vi "ECSv1_12.vi"() -> ()   [LabVIEW 2018]
uses:
  <vilib>/sound2/lvsound2.llb/Sampling Mode.ctl
  <vilib>/sound2/lvsound2.llb/Sound Data Format.ctl
  <vilib>/DAQmx/write.llb/DAQmx Write (Analog 1D DBL 1Chan NSamp).vi
  <vilib>/DAQmx/write.llb/DAQmx Write (Analog Wfm 1Chan NSamp).vi
  <vilib>/DAQmx/write.llb/DAQmx Write (Digital Bool 1Line 1Point).vi
  <vilib>/DAQmx/read.llb/DAQmx Read (Analog 1D Wfm NChan NSamp).vi
  <vilib>/DAQmx/create/channels.llb/DAQmx Create Channel (AI-Voltage-Basic).vi
  <vilib>/DAQmx/configure/timing.llb/DAQmx Timing (Sample Clock).vi
  <vilib>/sound2/lvsound2.llb/Sound File Write Open.vi
  <vilib>/sound2/lvsound2.llb/Sound Input Read (DBL).vi
  <vilib>/measure/maspectr.llb/FFT Power Spectral Density for N Chan.vi
  <vilib>/sound2/lvsound2.llb/Sound File Write (DBL).vi
  <vilib>/DAQmx/create/channels.llb/DAQmx Create Channel (DO-Digital Output).vi
  <vilib>/DAQmx/miscellaneous.llb/DAQmx Fill In Error Info.vi
  <vilib>/DAQmx/create/channels.llb/DAQmx Create Channel (CO-Pulse Generation-Time).vi
  <vilib>/DAQmx/configure/timing.llb/DAQmx Timing (Implicit).vi
  <vilib>/DAQmx/create/channels.llb/DAQmx Create Channel (AO-Voltage-Basic).vi
  <vilib>/DAQmx/configure/timing.llb/DAQmx Timing (Use Waveform).vi
  <vilib>/ptbypt/NI_PtbyPt.lvlib
  <vilib>/measure/NI_MAPro.lvlib
  <vilib>/measure/NI_MABase.lvlib
panel:
  in  "Flash Amp (V)":dbl=5.0 step=0.25
  in  "Flash Dur (s)":dbl=0.5 step=0.1
  in  "Single Flash":bool
  in  "LED Stim Channel":tag="Dev1/ao1"
  in  "LED OFF":bool
  in  "CoAx LED":bool
  in  "Enable Stim":bool=TRUE
  out "Numeric":i32
  out "x/y":dbl
  in  "Twin Pulse":bool
  out "EEG Chart":dynamicdata(graph)
  in  "Safety Duration":u32=250
  in  "Stim Safety":tag="Dev1/port0/line3"
  in  "Mic Ch":dbl
  in  "Vid  Synch":tag="Dev1/port1/line3"
  in  "Vid Synch":bool=TRUE
  in  "Air Puff Train":bool
  in  "Puff Interval (s)":dbl=0.5
  out "Puff Count":i32
  in  "Train Duration (s)":dbl=5.0
  in  "Air Puff":bool
  in  "Air Puff Channel":tag="Dev1/port0/line2"
  in  "Air Puff \nDuration (ms)":u32=500
  in  "Pause Dur":dbl=4.0
  out "Microphone Periodogram":cluster{"f0":dbl, "df":dbl, "magnitude":dbl[]}[](graph)
  out "Freq (Hz)":i32
  out "Stim":bool
  in  "Follow Freq\nStart":bool
  in  "Record Sound":bool=TRUE
  out "Sound File":path
  in  "Line ID":string
  in  "Ch 3. Name/Disc":string="None"
  in  "Ch 2. Name/Disc":string="L_DLM"
  in  "Ch 1. Name/Disc":string="None"
  in  "Show Triggered Response":bool=TRUE
  in  "Single Pulse":bool
  in  "Burst\nStart":bool
  out "Stimulation Chart":dynamicdata(graph)
  in  "Comments":string
  in  "Pulse Amp. (V)":dbl step=10.0
  in  "Age":dbl
  in  "Sex":string
  in  "Genotype":string
  in  "Operator":string="Atulya Iyengar"
  in  "Proposed Filename":path
  out "Trace File":path
  out "Recording":bool
  in  "Record":bool
  in  "Test Freq (Hz)":dbl
  in  "Test Dur (s)":dbl
  in  "Burst Freq (Hz)":dbl
  in  "Burst Dur (s)":dbl
  in  "Stimulator Trigger Channel":tag="Dev1/ctr0"
  in  "Burst/Test\nStart":bool
  out "Waveform Graph":dynamicdata(graph)=[{"t0"=timestamp(3548164212.270314 s since 1904-01-01), "dt"=4.999999999999997e-05, "Y"=[], "attributes"=variant("NI_ChannelName"=variant(string "Dev1/ai1"), "NI_UnitDescription"=variant(string "Volts"))}, {"t0"=timestamp(3548164212.2703266 s since 1904-01-01), "dt"=4.999999999999997e-05, "Y"=[], "attributes"=variant("NI_ChannelName"=variant(string "Dev1/ai2"), "NI_UnitDescription"=variant(string "Volts"))}, {"t0"=timestamp(3548164212.270339 s since 1904-01-01), "dt"=4.999999999999997e-05, "Y"=[], "attributes"=variant("NI_ChannelName"=variant(string "Dev1/ai3"), "NI_UnitDescription"=variant(string "Volts"))}]
  out "DLM Chart":dynamicdata(graph)
  in  "Buffer Size":i32=8000
  in  "stop":bool
  in  "Sampling Rate":dbl=20000.0 format="%0.2f"
  in  "AI Channels":tag="Dev1/ai1:4, Dev1/ai7, Dev1/ai5"
  # "ECS Control Panel\nversion: 1.12"
  # "Created by \nAtulya Iyengar 2019"
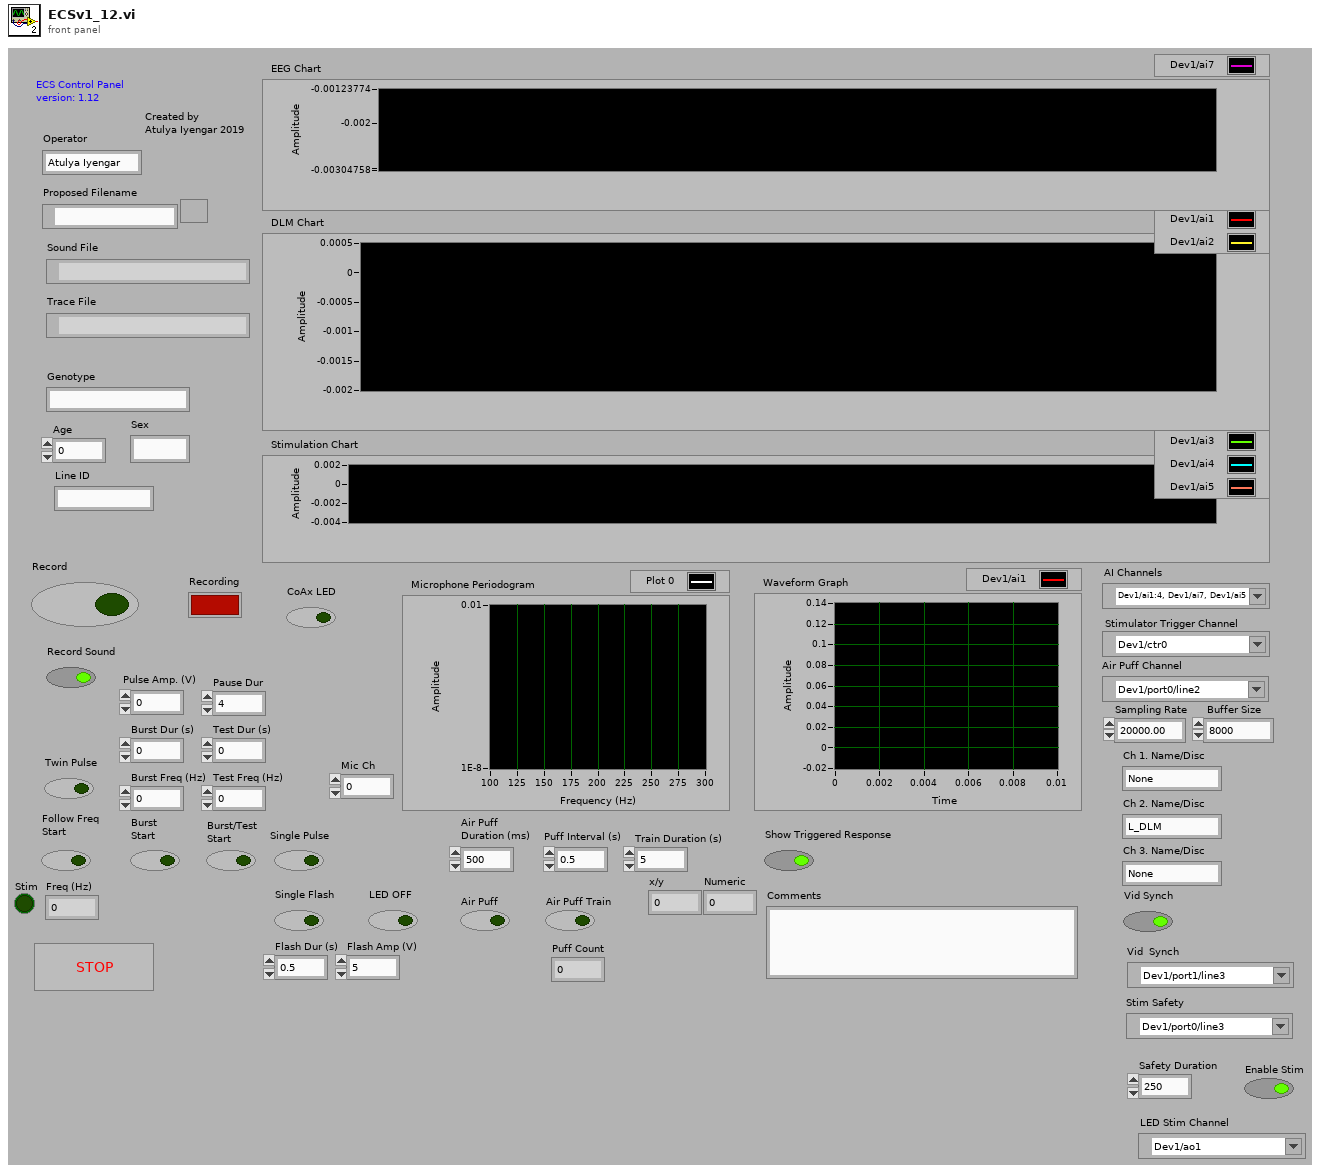
[diagram p1: front panel]
types:
  T1 = enum16{"Sine Wave", "Triangle Wave", "Square Wave", "Sawtooth Wave"}
  T2 = cluster{"averaging mode":enum16{"No averaging", "Vector averaging", "RMS averaging", "Peak hold"}, "weighting mode":enum16{"Linear", "Exponential"}, "number of averages":u32}
  T3 = typedef "Sound Data Format.ctl" = cluster{"sample rate (S/s)":dbl, "number of channels":i32, "bits per sample":i32}
  T4 = typedef "Sampling Mode.ctl" = i32
  T5 = typedef "Sound File Refnum.ctl" = refnum<file>
  T6 = typedef "Sound Input Task ID.ctl" = u32
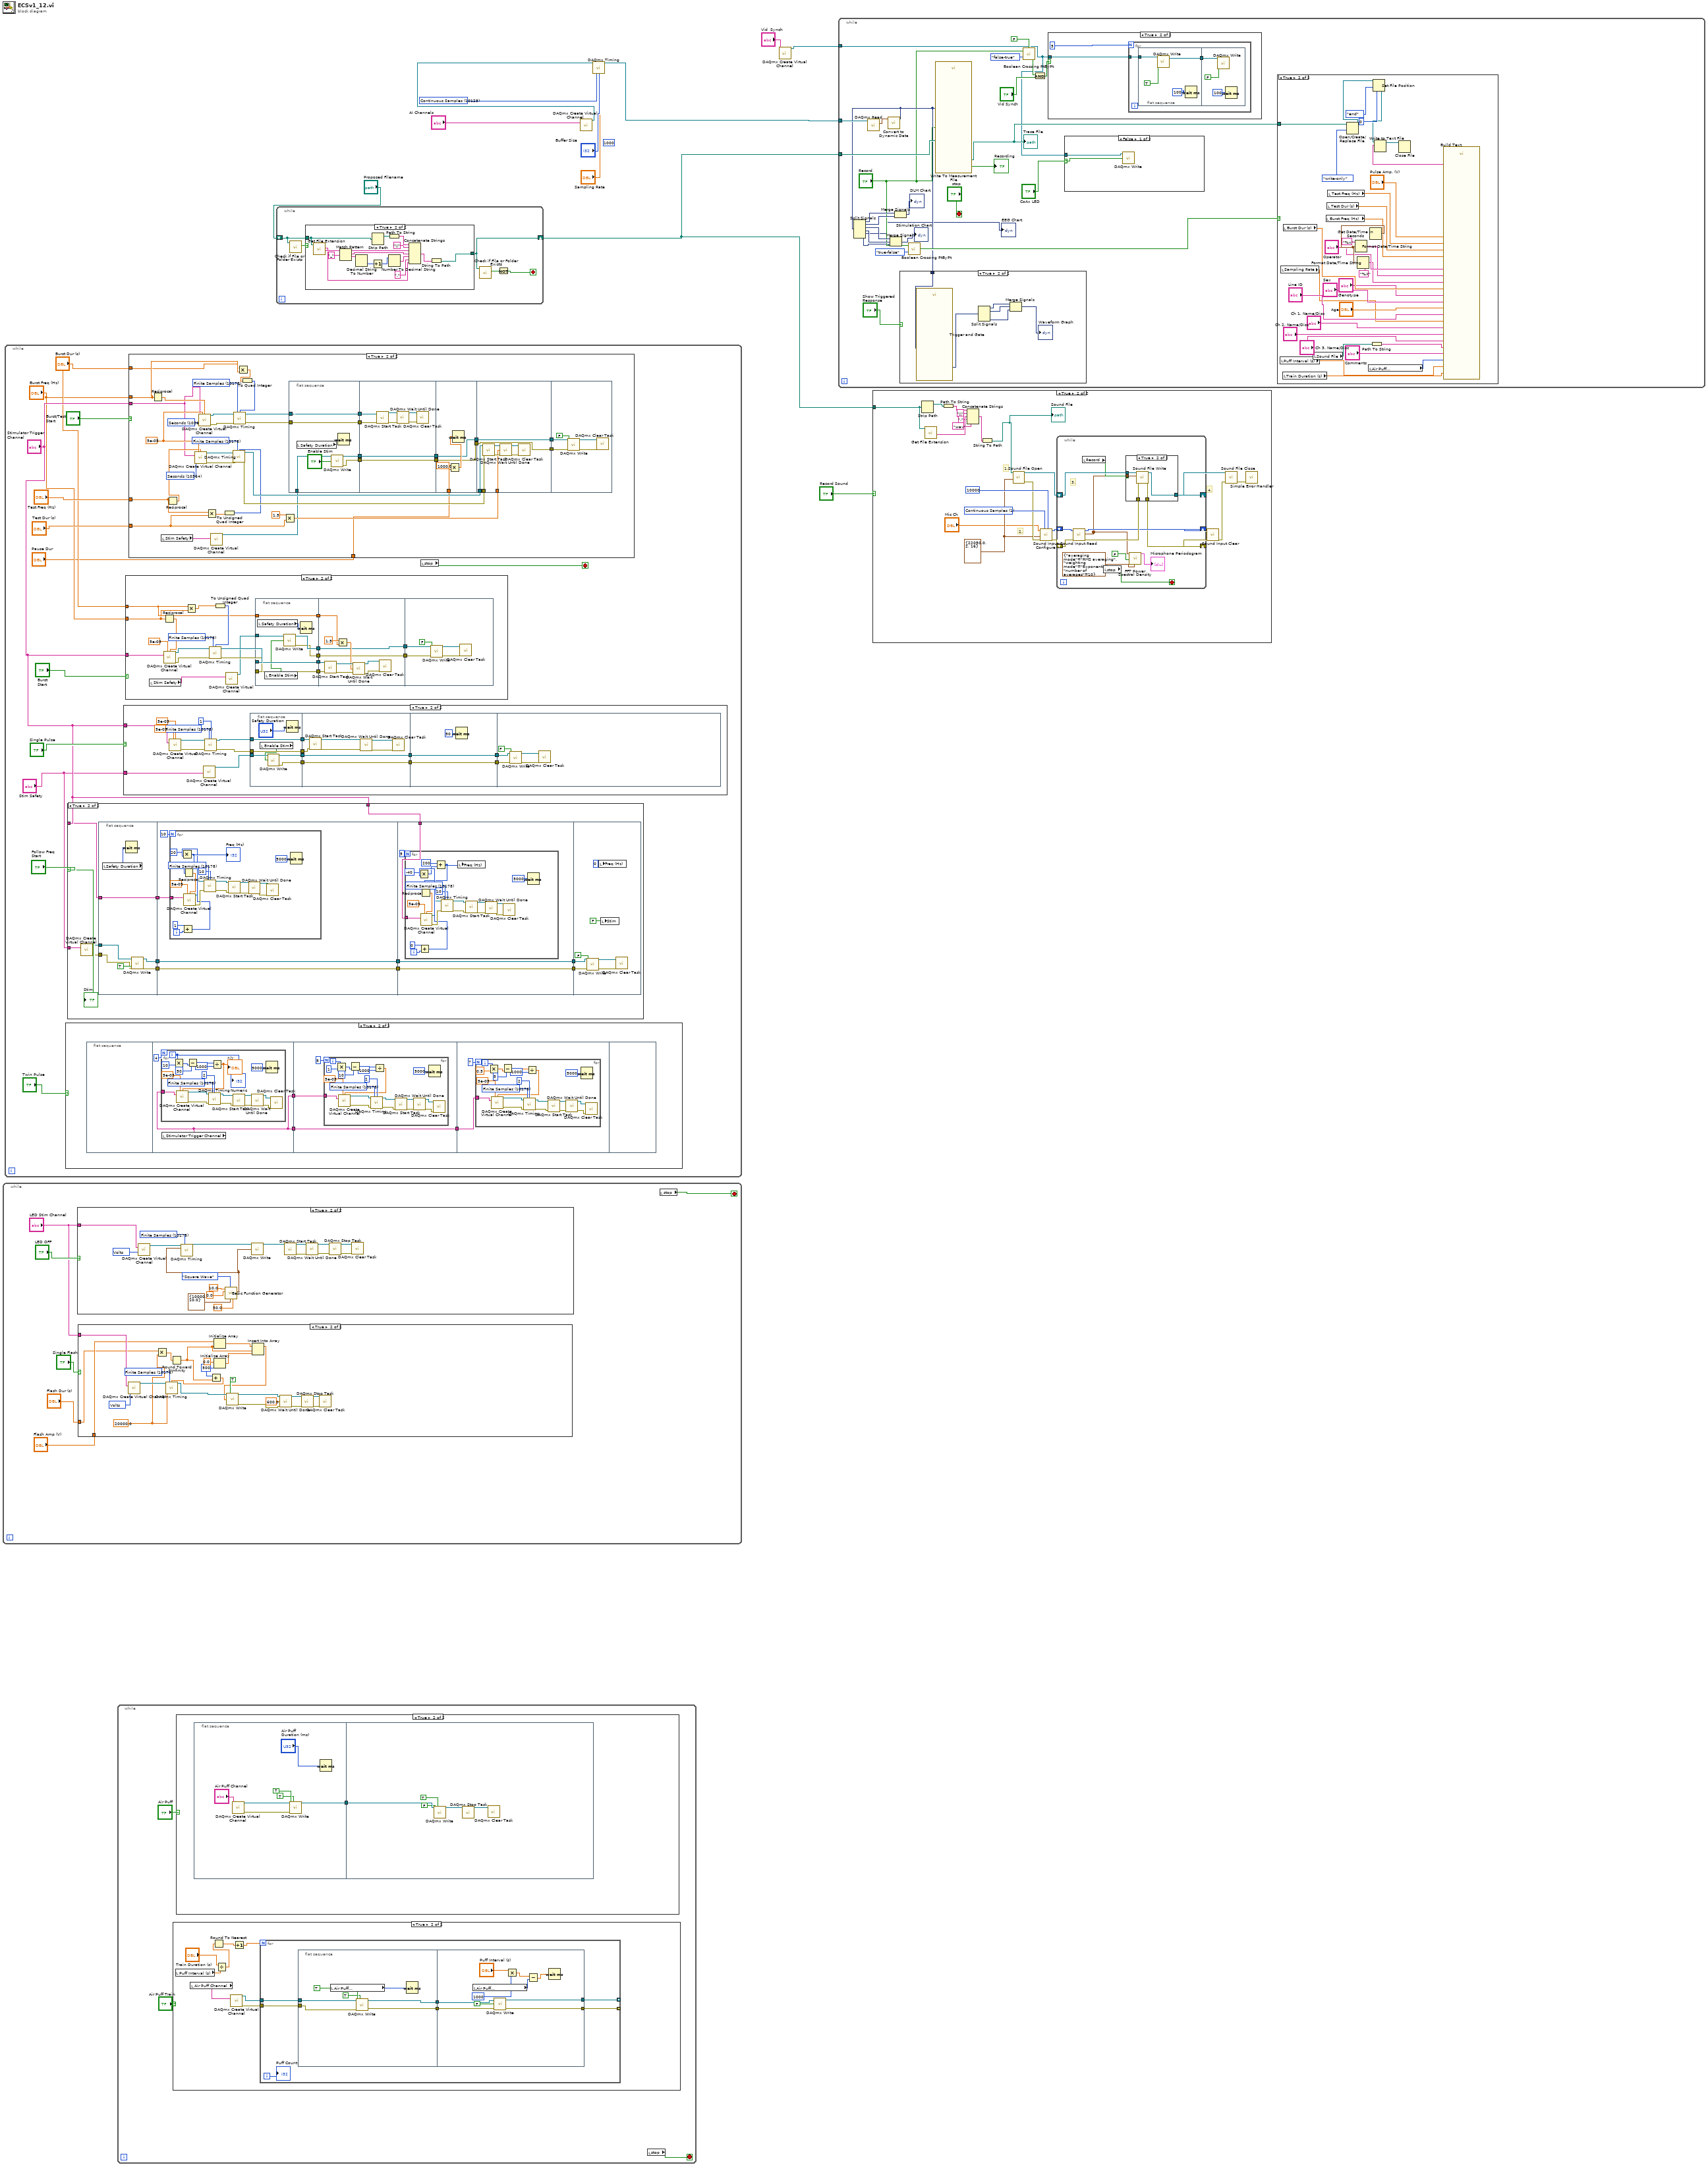
[diagram p0: block diagram]
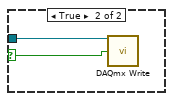
[diagram p14: hidden frame]
diagram:
  (unwired) 1000 ("samples per channel")
  w10 = 10123 items=["Finite Samples"=10178, "Continuous Samples"=10123, "Hardware Timed Single Point"=12522] ("sample mode")
  n1 = while {
    stop <- w17 stop-if-true
    n2 = case shown="True" "LED OFF" {
      tunnel: "LED Stim Channel" -> [_ w42]
      frame False {
      }
      frame True {
        w57 = 10178 items=["Finite Samples"=10178, "Continuous Samples"=10123, "Hardware Timed Single Point"=12522] ("sample mode")
        w59 = 10348 items=["Volts"=10348, "From Custom Scale"=10065] ("units")
        n3 = call-poly <vilib>:"DAQmx Create Virtual Channel.vi"("physical channels"=w42, "units"=w59) -> ("task out"=w58:refnum<k21>)  [unwired: 12 in, 1 out]
        n4 = call <vilib>:"Basic Function Generator.vi"("square wave duty cycle (%)"=50.0, "sampling info"=cluster{"Fs":dbl, "#s":dbl} {"Fs"=10000.0, "#s"=10.0}, "signal type"=T1."Square Wave", "amplitude"=0.0, "frequency"=10.0) -> ("signal out"=w52:waveform(dbl))  [unwired: 4 in, 2 out]
        n5 = call-poly <vilib>:"DAQmx Timing.vi"("task/channels in"=w58, "sample mode"=w57, "waveform"=w52) -> ("task out"=w53:refnum<k21>)  [unwired: 11 in, 1 out]
        n6 = call-poly <vilib>:"DAQmx Write.vi"("task/channels in"=w53, "data"=w52) -> ("task out"=w51:refnum<k21>)  [unwired: 11 in, 2 out]
        n7 = call <vilib>:"DAQmx Start Task.vi"("task/channels in"=w51) -> ("task out"=w50:refnum<k21>, "error out"=w49:errorcluster)  [unwired: 13 in]
        n8 = call <vilib>:"DAQmx Wait Until Done.vi"("task/channels in"=w50, "error in"=w49) -> ("task out"=w48:refnum<k21>, "error out"=w47:errorcluster)  [unwired: 12 in]
        n9 = call <vilib>:"DAQmx Stop Task.vi"("task/channels in"=w48, "error in"=w47) -> ("task out"=w46:refnum<k21>, "error out"=w45:errorcluster)  [unwired: 12 in]
        n10 = call <vilib>:"DAQmx Clear Task.vi"("task in"=w46, "error in"=w45) -> ()  [unwired: 13 in, 1 out]
      }
    }
    n11 = case shown="True" "Single Flash" {
      tunnel: "Flash Amp (V)" -> [_ w37]
      tunnel: "LED Stim Channel" -> [_ w41]
      tunnel: "Flash Dur (s)" -> [_ w36]
      frame False {
      }
      frame True {
        w30 = 500 ("dimension size")
        w38 = 10178 items=["Finite Samples"=10178, "Continuous Samples"=10123, "Hardware Timed Single Point"=12522] ("sample mode")
        w35 = 20000.0 ("rate")
        w40 = 10348 items=["Volts"=10348, "From Custom Scale"=10065] ("units")
        n12 = call-poly <vilib>:"DAQmx Create Virtual Channel.vi"("physical channels"=w41, "units"=w40) -> ("task out"=w39:refnum<k21>)  [unwired: 12 in, 1 out]
        n13 = Multiply(x=w36, y=w35) -> (x*y=w34:dbl)
        n14 = Round Toward +Infinity(x=w34) -> (ceil(x): smallest int >= x=w29:dbl)
        n15 = Add(x=w30, y=w29) -> (x+y=w28:dbl)
        n16 = call-poly <vilib>:"DAQmx Timing.vi"("task/channels in"=w39, "sample mode"=w38, "samples per channel"=w28, "rate"=w35) -> ("task out"=w27:refnum<k21>)  [unwired: 10 in, 1 out]
        n17 = Initialize Array(w37, w29) -> (w32:dbl[])
        n18 = Initialize Array(0.0 ("element"), w30) -> (w31:dbl[])
        n19 = Insert Into Array(array=w32, index=w29, new element=w31) -> (w25:dbl[])
        n20 = call-poly <vilib>:"DAQmx Write.vi"("task/channels in"=w27, "auto start"=TRUE, "data"=w25) -> ("task out"=w23:refnum<k21>, "error out"=w22:errorcluster)  [unwired: 10 in, 1 out]
        n21 = call <vilib>:"DAQmx Wait Until Done.vi"("task/channels in"=w23, "timeout (sec)"=600.0, "error in"=w22) -> ("task out"=w21:refnum<k21>, "error out"=w20:errorcluster)  [unwired: 11 in]
        n22 = call <vilib>:"DAQmx Stop Task.vi"("task/channels in"=w21, "error in"=w20) -> ("task out"=w19:refnum<k21>, "error out"=w18:errorcluster)  [unwired: 12 in]
        n23 = call <vilib>:"DAQmx Clear Task.vi"("task in"=w19, "error in"=w18) -> ()  [unwired: 13 in, 1 out]
      }
    }
    n24 = local read "stop"() -> (w17:bool)
  }
  n25 = while {
    stop <- w71 stop-if-true
    n26 = case shown="True" "Twin Pulse" {
      frame False {
      }
      frame True {
        n27 = flat-sequence {
          tunnel: [w76] -> w75
          tunnel: [w76] -> w74
          tunnel: w75 -> [w100]
          tunnel: w74 -> [w98]
          tunnel: [w98] -> w73
          tunnel: w73 -> [w121]
          frame #0 {
          }
          frame #1 {
            n28 = local read "Stimulator Trigger Channel"() -> (w76:tag)
            n29 = for {
              N: 4 -> [_]
              tunnel: w76 -> [w90]
              i -> [w78]
              w96 = 10178 items=["Finite Samples"=10178, "Continuous Samples"=10123, "Hardware Timed Single Point"=12522] ("sample mode")
              n30 = Multiply(x=w78, y=10) -> (x*y=w92:i32)
              n31 = Subtract(x=50, y=w92) -> (x-y=w86:i32)
              n32 = Divide(x=w86, y=1000) -> (x/y=w84:dbl)
              "x/y" <- w84
              n33 = call-poly <vilib>:"DAQmx Create Virtual Channel.vi"("high time"=5e-05, "low time"=w84, "counter"=w90) -> ("task out"=w89:refnum<k21>, "error out"=w88:errorcluster)  [unwired: 6 in, 5 out]
              n34 = call-poly <vilib>:"DAQmx Timing.vi"("task/channels in"=w89, "sample mode"=w96, "samples per channel"=2, "error in"=w88) -> ("task out"=w87:refnum<k21>, "error out"=w97:errorcluster)  [unwired: 10 out]
              n35 = call <vilib>:"DAQmx Start Task.vi"("task/channels in"=w87, "error in"=w97) -> ("task out"=w79:refnum<k21>, "error out"=w80:errorcluster)  [unwired: 12 out]
              n36 = call <vilib>:"DAQmx Wait Until Done.vi"("task/channels in"=w79, "error in"=w80) -> ("task out"=w82:refnum<k21>, "error out"=w81:errorcluster)  [unwired: 1 in, 11 out]
              n37 = Wait (ms)(milliseconds to wait=u32 5000) -> ()  [unwired: 1 out]
              n38 = call <vilib>:"DAQmx Clear Task.vi"("task in"=w82, "error in"=w81) -> ()  [unwired: 14 out]
              "Numeric" <- w78
            }
          }
          frame #2 {
            n39 = for {
              N: 5 -> [_]
              tunnel: w100 -> [w103]
              i -> [w101]
              w119 = 10178 items=["Finite Samples"=10178, "Continuous Samples"=10123, "Hardware Timed Single Point"=12522] ("sample mode")
              n40 = Multiply(x=w101, y=1) -> (x*y=w115:i32)
              n41 = Subtract(x=10, y=w115) -> (x-y=w110:i32)
              n42 = Divide(x=w110, y=1000) -> (x/y=w102:dbl)
              n43 = call-poly <vilib>:"DAQmx Create Virtual Channel.vi"("high time"=5e-05, "low time"=w102, "counter"=w103) -> ("task out"=w113:refnum<k21>, "error out"=w112:errorcluster)  [unwired: 6 in, 5 out]
              n44 = call-poly <vilib>:"DAQmx Timing.vi"("task/channels in"=w113, "sample mode"=w119, "samples per channel"=2, "error in"=w112) -> ("task out"=w111:refnum<k21>, "error out"=w120:errorcluster)  [unwired: 10 out]
              n45 = call <vilib>:"DAQmx Start Task.vi"("task/channels in"=w111, "error in"=w120) -> ("task out"=w104:refnum<k21>, "error out"=w105:errorcluster)  [unwired: 12 out]
              n46 = call <vilib>:"DAQmx Wait Until Done.vi"("task/channels in"=w104, "error in"=w105) -> ("task out"=w107:refnum<k21>, "error out"=w106:errorcluster)  [unwired: 1 in, 11 out]
              n47 = Wait (ms)(milliseconds to wait=u32 5000) -> ()  [unwired: 1 out]
              n48 = call <vilib>:"DAQmx Clear Task.vi"("task in"=w107, "error in"=w106) -> ()  [unwired: 14 out]
            }
          }
          frame #3 {
            n49 = for {
              N: 7 -> [_]
              tunnel: w121 -> [w126]
              i -> [w123]
              w141 = 10178 items=["Finite Samples"=10178, "Continuous Samples"=10123, "Hardware Timed Single Point"=12522] ("sample mode")
              n50 = Multiply(x=w123, y=0.5) -> (x*y=w138:dbl)
              n51 = Subtract(x=5, y=w138) -> (x-y=w133:dbl)
              n52 = Divide(x=w133, y=1000) -> (x/y=w125:dbl)
              n53 = call-poly <vilib>:"DAQmx Create Virtual Channel.vi"("high time"=5e-05, "low time"=w125, "counter"=w126) -> ("task out"=w136:refnum<k21>, "error out"=w135:errorcluster)  [unwired: 6 in, 5 out]
              n54 = call-poly <vilib>:"DAQmx Timing.vi"("task/channels in"=w136, "sample mode"=w141, "samples per channel"=2, "error in"=w135) -> ("task out"=w134:refnum<k21>, "error out"=w142:errorcluster)  [unwired: 10 out]
              n55 = call <vilib>:"DAQmx Start Task.vi"("task/channels in"=w134, "error in"=w142) -> ("task out"=w127:refnum<k21>, "error out"=w128:errorcluster)  [unwired: 12 out]
              n56 = call <vilib>:"DAQmx Wait Until Done.vi"("task/channels in"=w127, "error in"=w128) -> ("task out"=w130:refnum<k21>, "error out"=w129:errorcluster)  [unwired: 1 in, 11 out]
              n57 = Wait (ms)(milliseconds to wait=u32 5000) -> ()  [unwired: 1 out]
              n58 = call <vilib>:"DAQmx Clear Task.vi"("task in"=w130, "error in"=w129) -> ()  [unwired: 14 out]
            }
          }
          frame #4 {
          }
        }
      }
    }
    n59 = case shown="True" "Follow Freq\nStart" {
      selector: "Follow Freq\nStart" -> [_ w155]
      tunnel: "Stimulator Trigger Channel" -> [_ w154]
      tunnel: "Stimulator Trigger Channel" -> [_ w153]
      tunnel: "Stim Safety" -> [_ w151]
      frame False {
      }
      frame True {
        n60 = call-poly <vilib>:"DAQmx Create Virtual Channel.vi"("lines"=w151) -> ("task out"=w150:refnum<k21>, "error out"=w149:errorcluster)  [unwired: 4 in, 9 out]
        n61 = flat-sequence {
          tunnel: w154 -> [w162]
          tunnel: [w162] -> w152
          tunnel: w150 -> [w159]
          tunnel: w149 -> [w158]
          tunnel: [w157] -> w146
          tunnel: [w156] -> w145
          tunnel: w152 -> [w165]
          tunnel: [w164] -> w147
          tunnel: w146 -> [w164]
          tunnel: w145 -> [w163]
          tunnel: [w163] -> w144
          tunnel: w153 -> [w188]
          tunnel: [w187] -> w148
          tunnel: w147 -> [w187]
          tunnel: w144 -> [w186]
          tunnel: [w186] -> w143
          tunnel: w148 -> [w212]
          tunnel: w143 -> [w211]
          frame #0 {
            n62 = local read "Safety Duration"() -> (w160:u32)
            n63 = Wait (ms)(milliseconds to wait=w160) -> ()  [unwired: 1 out]
            n64 = call-poly <vilib>:"DAQmx Write.vi"("task/channels in"=w159, "data"=TRUE, "error in"=w158) -> ("task out"=w157:refnum<k21>, "error out"=w156:errorcluster)  [unwired: 1 in, 10 out]
          }
          frame #1 {
            n65 = for {
              N: 10 -> [_]
              tunnel: w165 -> [w177]
              i -> [w175]
              w169 = 10178 items=["Finite Samples"=10178, "Continuous Samples"=10123, "Hardware Timed Single Point"=12522] ("sample mode")
              n66 = Add(x=1, y=w175) -> (x+y=w172:i32)
              n67 = Multiply(x=20, y=w172) -> (x*y=w173:i32)
              "Freq (Hz)" <- w173
              n68 = Reciprocal(x=w173) -> (1/x=w176:dbl)
              n69 = call-poly <vilib>:"DAQmx Create Virtual Channel.vi"("high time"=5e-05, "low time"=w176, "counter"=w177) -> ("task out"=w167:refnum<k21>, "error out"=w185:errorcluster)  [unwired: 6 in, 5 out]
              n70 = call-poly <vilib>:"DAQmx Timing.vi"("task/channels in"=w167, "sample mode"=w169, "samples per channel"=10, "error in"=w185) -> ("task out"=w184:refnum<k21>, "error out"=w183:errorcluster)  [unwired: 10 out]
              n71 = call <vilib>:"DAQmx Start Task.vi"("task/channels in"=w184, "error in"=w183) -> ("task out"=w180:refnum<k21>, "error out"=w179:errorcluster)  [unwired: 12 out]
              n72 = call <vilib>:"DAQmx Wait Until Done.vi"("task/channels in"=w180, "error in"=w179) -> ("task out"=w182:refnum<k21>, "error out"=w181:errorcluster)  [unwired: 1 in, 11 out]
              n73 = call <vilib>:"DAQmx Clear Task.vi"("task in"=w182, "error in"=w181) -> ()  [unwired: 14 out]
              n74 = Wait (ms)(milliseconds to wait=u32 5000) -> ()  [unwired: 1 out]
            }
          }
          frame #2 {
            n75 = for {
              N: 5 -> [_]
              tunnel: w188 -> [w190]
              i -> [w201]
              w196 = 10178 items=["Finite Samples"=10178, "Continuous Samples"=10123, "Hardware Timed Single Point"=12522] ("sample mode")
              n76 = Add(x=0, y=w201) -> (x+y=w199:i32)
              n77 = Multiply(x=-40, y=w199) -> (x*y=w193:i32)
              n78 = Add(x=200, y=w193) -> (x+y=w191:i32)
              n79 = Reciprocal(x=w191) -> (1/x=w202:dbl)
              n80 = call-poly <vilib>:"DAQmx Create Virtual Channel.vi"("high time"=5e-05, "low time"=w202, "counter"=w190) -> ("task out"=w194:refnum<k21>, "error out"=w210:errorcluster)  [unwired: 6 in, 5 out]
              n81 = call-poly <vilib>:"DAQmx Timing.vi"("task/channels in"=w194, "sample mode"=w196, "samples per channel"=10, "error in"=w210) -> ("task out"=w209:refnum<k21>, "error out"=w208:errorcluster)  [unwired: 10 out]
              n82 = local write "Freq (Hz)"(w191) -> ()
              n83 = call <vilib>:"DAQmx Start Task.vi"("task/channels in"=w209, "error in"=w208) -> ("task out"=w205:refnum<k21>, "error out"=w204:errorcluster)  [unwired: 12 out]
              n84 = call <vilib>:"DAQmx Wait Until Done.vi"("task/channels in"=w205, "error in"=w204) -> ("task out"=w207:refnum<k21>, "error out"=w206:errorcluster)  [unwired: 1 in, 11 out]
              n85 = call <vilib>:"DAQmx Clear Task.vi"("task in"=w207, "error in"=w206) -> ()  [unwired: 14 out]
              n86 = Wait (ms)(milliseconds to wait=u32 5000) -> ()  [unwired: 1 out]
            }
          }
          frame #3 {
            n87 = call-poly <vilib>:"DAQmx Write.vi"("task/channels in"=w212, "data"=FALSE, "error in"=w211) -> ("task out"=w214:refnum<k21>, "error out"=w213:errorcluster)  [unwired: 1 in, 10 out]
            n88 = local write "Freq (Hz)"(0 ("Freq (Hz)")) -> ()
            n89 = local write "Stim"(FALSE ("Stim")) -> ()
            n90 = call <vilib>:"DAQmx Clear Task.vi"("task in"=w214, "error in"=w213) -> ()  [unwired: 14 out]
          }
        }
        "Stim" <- w155
      }
    }
    n91 = case shown="True" "Single Pulse" {
      tunnel: "Stimulator Trigger Channel" -> [_ w236]
      tunnel: "Stim Safety" -> [_ w222]
      frame False {
      }
      frame True {
        w233 = 10178 items=["Finite Samples"=10178, "Continuous Samples"=10123, "Hardware Timed Single Point"=12522] ("sample mode")
        n92 = call-poly <vilib>:"DAQmx Create Virtual Channel.vi"("high time"=5e-05, "low time"=5e-05, "counter"=w236) -> ("task out"=w234:refnum<k21>, "error out"=w231:errorcluster)  [unwired: 6 in, 5 out]
        n93 = call-poly <vilib>:"DAQmx Create Virtual Channel.vi"("lines"=w222) -> ("task out"=w225:refnum<k21>)  [unwired: 4 in, 10 out]
        n94 = call-poly <vilib>:"DAQmx Timing.vi"("task/channels in"=w234, "sample mode"=w233, "samples per channel"=1, "error in"=w231) -> ("task out"=w230:refnum<k21>, "error out"=w229:errorcluster)  [unwired: 10 out]
        n95 = flat-sequence {
          tunnel: w229 -> [w242]
          tunnel: w230 -> [w243]
          tunnel: [w243] -> w227
          tunnel: [w242] -> w226
          tunnel: w225 -> [w241]
          tunnel: [w240] -> w224
          tunnel: [w239] -> w223
          tunnel: w227 -> [w251]
          tunnel: w226 -> [w250]
          tunnel: w224 -> [w245]
          tunnel: [w245] -> w221
          tunnel: w223 -> [w244]
          tunnel: [w244] -> w219
          tunnel: w221 -> [w254]
          tunnel: [w254] -> w220
          tunnel: w219 -> [w253]
          tunnel: [w253] -> w218
          tunnel: w220 -> [w259]
          tunnel: w218 -> [w255]
          frame #0 {
            n96 = local read "Enable Stim"() -> (w237:bool)
            n97 = call-poly <vilib>:"DAQmx Write.vi"("task/channels in"=w241, "data"=w237) -> ("task out"=w240:refnum<k21>, "error out"=w239:errorcluster)  [unwired: 2 in, 10 out]
            n98 = Wait (ms)(milliseconds to wait="Safety Duration") -> ()  [unwired: 1 out]
          }
          frame #1 {
            n99 = call <vilib>:"DAQmx Start Task.vi"("task/channels in"=w251, "error in"=w250) -> ("task out"=w249:refnum<k21>, "error out"=w248:errorcluster)  [unwired: 12 out]
            n100 = call <vilib>:"DAQmx Wait Until Done.vi"("task/channels in"=w249, "error in"=w248) -> ("task out"=w247:refnum<k21>, "error out"=w246:errorcluster)  [unwired: 1 in, 11 out]
            n101 = call <vilib>:"DAQmx Clear Task.vi"("task in"=w247, "error in"=w246) -> ()  [unwired: 14 out]
          }
          frame #2 {
            n102 = Wait (ms)(milliseconds to wait=u32 50) -> ()  [unwired: 1 out]
          }
          frame #3 {
            n103 = call-poly <vilib>:"DAQmx Write.vi"("task/channels in"=w259, "data"=FALSE, "error in"=w255) -> ("task out"=w257:refnum<k21>, "error out"=w256:errorcluster)  [unwired: 1 in, 10 out]
            n104 = call <vilib>:"DAQmx Clear Task.vi"("task in"=w257, "error in"=w256) -> ()  [unwired: 14 out]
          }
        }
      }
    }
    n105 = case shown="True" "Burst\nStart" {
      tunnel: "Burst Freq (Hz)" -> [_ w269]
      tunnel: "Burst Dur (s)" -> [_ w273]
      tunnel: "Stimulator Trigger Channel" -> [_ w270]
      frame False {
      }
      frame True {
        w276 = 10178 items=["Finite Samples"=10178, "Continuous Samples"=10123, "Hardware Timed Single Point"=12522] ("sample mode")
        n106 = local read "Stim Safety"() -> (w265:tag)
        n107 = Reciprocal(x=w269) -> (1/x=w279:dbl)
        n108 = call-poly <vilib>:"DAQmx Create Virtual Channel.vi"("high time"=5e-05, "low time"=w279, "counter"=w270) -> ("task out"=w275:refnum<k21>, "error out"=w272:errorcluster)  [unwired: 6 in, 5 out]
        n109 = Multiply(x=w273, y=w269) -> (x*y=w278:dbl)
        n110 = To Unsigned Quad Integer(1:w278) -> (0:w277:u64)
        n111 = call-poly <vilib>:"DAQmx Timing.vi"("task/channels in"=w275, "sample mode"=w276, "samples per channel"=w277, "error in"=w272) -> ("task out"=w274:refnum<k21>, "error out"=w271:errorcluster)  [unwired: 10 out]
        n112 = call-poly <vilib>:"DAQmx Create Virtual Channel.vi"("lines"=w265) -> ("task out"=w264:refnum<k21>)  [unwired: 4 in, 10 out]
        n113 = flat-sequence {
          tunnel: w271 -> [w286]
          tunnel: w273 -> [w287]
          tunnel: w274 -> [w288]
          tunnel: [w288] -> w268
          tunnel: [w287] -> w267
          tunnel: [w286] -> w266
          tunnel: w264 -> [w284]
          tunnel: [w283] -> w263
          tunnel: [w282] -> w261
          tunnel: w268 -> [w299]
          tunnel: w267 -> [w295]
          tunnel: w266 -> [w293]
          tunnel: w263 -> [w290]
          tunnel: [w290] -> w262
          tunnel: w261 -> [w289]
          tunnel: [w289] -> w260
          tunnel: w262 -> [w301]
          tunnel: w260 -> [w300]
          frame #0 {
            n114 = local read "Safety Duration"() -> (w285:u32)
            n115 = local read "Enable Stim"() -> (w281:bool)
            n116 = call-poly <vilib>:"DAQmx Write.vi"("task/channels in"=w284, "data"=w281) -> ("task out"=w283:refnum<k21>, "error out"=w282:errorcluster)  [unwired: 2 in, 10 out]
            n117 = Wait (ms)(milliseconds to wait=w285) -> ()  [unwired: 1 out]
          }
          frame #1 {
            n118 = call <vilib>:"DAQmx Start Task.vi"("task/channels in"=w299, "error in"=w293) -> ("task out"=w298:refnum<k21>, "error out"=w292:errorcluster)  [unwired: 12 out]
            n119 = Multiply(x=1.5, y=w295) -> (x*y=w294:dbl)
            n120 = call <vilib>:"DAQmx Wait Until Done.vi"("task/channels in"=w298, "timeout (sec)"=w294, "error in"=w292) -> ("task out"=w297:refnum<k21>, "error out"=w291:errorcluster)  [unwired: 11 out]
            n121 = call <vilib>:"DAQmx Clear Task.vi"("task in"=w297, "error in"=w291) -> ()  [unwired: 14 out]
          }
          frame #2 {
            n122 = call-poly <vilib>:"DAQmx Write.vi"("task/channels in"=w301, "data"=FALSE, "error in"=w300) -> ("task out"=w303:refnum<k21>, "error out"=w302:errorcluster)  [unwired: 1 in, 10 out]
            n123 = call <vilib>:"DAQmx Clear Task.vi"("task in"=w303, "error in"=w302) -> ()  [unwired: 14 out]
          }
        }
      }
    }
    n124 = case shown="True" "Burst/Test\nStart" {
      tunnel: "Burst Freq (Hz)" -> [_ w322]
      tunnel: "Burst Dur (s)" -> [_ w321]
      tunnel: "Test Freq (Hz)" -> [_ w320]
      tunnel: "Test Dur (s)" -> [_ w319]
      tunnel: "Stimulator Trigger Channel" -> [_ w318]
      tunnel: "Pause Dur" -> [_ w317]
      frame False {
      }
      frame True {
        w329 = 5e-05 ("high time")
        w336 = 10364 items=["Seconds"=10364] ("units")
        w337 = 10364 items=["Seconds"=10364] ("units")
        w338 = 10178 items=["Finite Samples"=10178, "Continuous Samples"=10123, "Hardware Timed Single Point"=12522] ("sample mode")
        w339 = 10178 items=["Finite Samples"=10178, "Continuous Samples"=10123, "Hardware Timed Single Point"=12522] ("sample mode")
        n125 = Reciprocal(x=w322) -> (1/x=w328:dbl)
        n126 = local read "Stim Safety"() -> (w305:tag)
        n127 = Reciprocal(x=w320) -> (1/x=w327:dbl)
        n128 = call-poly <vilib>:"DAQmx Create Virtual Channel.vi"("high time"=w329, "low time"=w327, "counter"=w318, "units"=w336) -> ("task out"=w343:refnum<k21>, "error out"=w342:errorcluster)  [unwired: 5 in, 5 out]
        n129 = call-poly <vilib>:"DAQmx Create Virtual Channel.vi"("high time"=w329, "low time"=w328, "counter"=w318, "units"=w337) -> ("task out"=w341:refnum<k21>, "error out"=w340:errorcluster)  [unwired: 5 in, 5 out]
        n130 = Multiply(x=w320, y=w319) -> (x*y=w324:dbl)
        n131 = call-poly <vilib>:"DAQmx Create Virtual Channel.vi"("lines"=w305) -> ("task out"=w306:refnum<k21>)  [unwired: 4 in, 10 out]
        n132 = To Unsigned Quad Integer(1:w324) -> (0:w323:u64)
        n133 = call-poly <vilib>:"DAQmx Timing.vi"("task/channels in"=w343, "sample mode"=w339, "samples per channel"=w323, "error in"=w342) -> ("task out"=w334:refnum<k21>, "error out"=w333:errorcluster)  [unwired: 10 out]
        n134 = Multiply(x=w321, y=w322) -> (x*y=w326:dbl)
        n135 = To Quad Integer(1:w326) -> (0:w325:i64)
        n136 = call-poly <vilib>:"DAQmx Timing.vi"("task/channels in"=w341, "sample mode"=w338, "samples per channel"=w325, "error in"=w340) -> ("task out"=w335:refnum<k21>, "error out"=w332:errorcluster)  [unwired: 10 out]
        n137 = Multiply(x=1.5, y=w319) -> (x*y=w330:dbl)
        n138 = flat-sequence {
          tunnel: w332 -> [w349]
          tunnel: w335 -> [w350]
          tunnel: [w350] -> w316
          tunnel: [w349] -> w315
          tunnel: [w348] -> w311
          tunnel: [w347] -> w310
          tunnel: w306 -> [w345]
          tunnel: w316 -> [w354]
          tunnel: w315 -> [w353]
          tunnel: [w352] -> w312
          tunnel: w311 -> [w352]
          tunnel: w310 -> [w351]
          tunnel: [w351] -> w309
          tunnel: w317 -> [w363]
          tunnel: [w360] -> w313
          tunnel: w312 -> [w360]
          tunnel: w309 -> [w359]
          tunnel: [w359] -> w308
          tunnel: w334 -> [w368]
          tunnel: w333 -> [w367]
          tunnel: w330 -> [w366]
          tunnel: [w365] -> w314
          tunnel: w313 -> [w365]
          tunnel: w308 -> [w364]
          tunnel: [w364] -> w307
          tunnel: w314 -> [w374]
          tunnel: w307 -> [w373]
          frame #0 {
            n139 = local read "Safety Duration"() -> (w346:u32)
            n140 = call-poly <vilib>:"DAQmx Write.vi"("task/channels in"=w345, "data"="Enable Stim") -> ("task out"=w348:refnum<k21>, "error out"=w347:errorcluster)  [unwired: 2 in, 10 out]
            n141 = Wait (ms)(milliseconds to wait=w346) -> ()  [unwired: 1 out]
          }
          frame #1 {
            n142 = call <vilib>:"DAQmx Start Task.vi"("task/channels in"=w354, "error in"=w353) -> ("task out"=w358:refnum<k21>, "error out"=w357:errorcluster)  [unwired: 12 out]
            n143 = call <vilib>:"DAQmx Wait Until Done.vi"("task/channels in"=w358, "error in"=w357) -> ("task out"=w356:refnum<k21>, "error out"=w355:errorcluster)  [unwired: 1 in, 11 out]
            n144 = call <vilib>:"DAQmx Clear Task.vi"("task in"=w356, "error in"=w355) -> ()  [unwired: 14 out]
          }
          frame #2 {
            n145 = Multiply(x=1000.0, y=w363) -> (x*y=w361:dbl)
            n146 = Wait (ms)(milliseconds to wait=w361) -> ()  [unwired: 1 out]
          }
          frame #3 {
            n147 = call <vilib>:"DAQmx Start Task.vi"("task/channels in"=w368, "error in"=w367) -> ("task out"=w372:refnum<k21>, "error out"=w371:errorcluster)  [unwired: 12 out]
            n148 = call <vilib>:"DAQmx Wait Until Done.vi"("task/channels in"=w372, "timeout (sec)"=w366, "error in"=w371) -> ("task out"=w370:refnum<k21>, "error out"=w369:errorcluster)  [unwired: 11 out]
            n149 = call <vilib>:"DAQmx Clear Task.vi"("task in"=w370, "error in"=w369) -> ()  [unwired: 14 out]
          }
          frame #4 {
            n150 = call-poly <vilib>:"DAQmx Write.vi"("task/channels in"=w374, "data"=FALSE, "error in"=w373) -> ("task out"=w376:refnum<k21>, "error out"=w375:errorcluster)  [unwired: 1 in, 10 out]
            n151 = call <vilib>:"DAQmx Clear Task.vi"("task in"=w376, "error in"=w375) -> ()  [unwired: 14 out]
          }
        }
      }
    }
    n152 = local read "stop"() -> (w71:bool)
  }
  n153 = while {
    stop <- w378 stop-if-true
    n154 = case shown="True" "Air Puff Train" {
      frame False {
      }
      frame True {
        n155 = local read "Puff Interval (s)"() -> (w388:dbl)
        n156 = local read "Air Puff Channel"() -> (w385:tag)
        n157 = Divide(x="Train Duration (s)", y=w388) -> (x/y=w386:dbl)
        n158 = Round To Nearest(number=w386) -> (nearest integer value=w381:dbl)
        n159 = call-poly <vilib>:"DAQmx Create Virtual Channel.vi"("lines"=w385) -> ("task out"=w384:refnum<k21>, "error out"=w383:errorcluster)  [unwired: 4 in, 9 out]
        n160 = Increment(x=w381) -> (x+1=w382:dbl)
        n161 = for {
          N: w382 -> [_]
          tunnel: w384 -> [w394]
          tunnel: w383 -> [w393]
          tunnel: [w390] -> _ mode=indexing
          tunnel: [w389] -> _ mode=indexing
          i -> [w395]
          n162 = flat-sequence {
            tunnel: w394 -> [w401]
            tunnel: w393 -> [w400]
            tunnel: [w397] -> w392
            tunnel: [w396] -> w391
            tunnel: w392 -> [w407]
            tunnel: w391 -> [w405]
            tunnel: [w404] -> w390
            tunnel: [w403] -> w389
            frame #0 {
              n163 = local read "Air Puff \nDuration (ms)"() -> (w402:u32)
              n164 = call-poly <vilib>:"DAQmx Write.vi"("task/channels in"=w401, "auto start"=TRUE, "data"=TRUE, "error in"=w400) -> ("task out"=w397:refnum<k21>, "error out"=w396:errorcluster)  [unwired: 10 out]
              n165 = Wait (ms)(milliseconds to wait=w402) -> ()  [unwired: 1 out]
            }
            frame #1 {
              n166 = local read "Air Puff \nDuration (ms)"() -> (w412:u32)
              n167 = call-poly <vilib>:"DAQmx Write.vi"("task/channels in"=w407, "data"=FALSE, "error in"=w405) -> ("task out"=w404:refnum<k21>, "error out"=w403:errorcluster)  [unwired: 1 in, 10 out]
              n168 = Multiply(x="Puff Interval (s)", y=u32 1000) -> (x*y=w408:dbl)
              n169 = Subtract(x=w408, y=w412) -> (x-y=w411:dbl)
              n170 = Wait (ms)(milliseconds to wait=w411) -> ()  [unwired: 1 out]
            }
          }
          "Puff Count" <- w395
        }
      }
    }
    n171 = case shown="True" "Air Puff" {
      frame False {
      }
      frame True {
        n172 = flat-sequence {
          tunnel: [w416] -> w413
          tunnel: w413 -> [w425]
          frame #0 {
            n173 = call-poly <vilib>:"DAQmx Create Virtual Channel.vi"("lines"="Air Puff Channel") -> ("task out"=w419:refnum<k21>, "error out"=w418:errorcluster)  [unwired: 4 in, 9 out]
            n174 = call-poly <vilib>:"DAQmx Write.vi"("task/channels in"=w419, "auto start"=TRUE, "data"=TRUE, "error in"=w418) -> ("task out"=w416:refnum<k21>)  [unwired: 11 out]
            n175 = Wait (ms)(milliseconds to wait="Air Puff \nDuration (ms)") -> ()  [unwired: 1 out]
          }
          frame #1 {
            n176 = call-poly <vilib>:"DAQmx Write.vi"("task/channels in"=w425, "auto start"=TRUE, "data"=FALSE) -> ("task out"=w422:refnum<k21>)  [unwired: 1 in, 11 out]
            n177 = call <vilib>:"DAQmx Stop Task.vi"("task/channels in"=w422) -> ("task out"=w421:refnum<k21>)  [unwired: 1 in, 13 out]
            n178 = call <vilib>:"DAQmx Clear Task.vi"("task in"=w421) -> ()  [unwired: 1 in, 14 out]
          }
        }
      }
    }
    n179 = local read "stop"() -> (w378:bool)
  }
  n180 = while {
    shift-right: [w428] -> w4
    shift-left: "Proposed Filename" -> [w430]
    stop <- w426 stop-if-true
    n181 = call <vilib>:"Check if File or Folder Exists.vi"("path"=w430) -> ("file or folder exists?"=w429:bool)  [unwired: 1 in, 9 out]
    n182 = case shown="True" w429 {
      tunnel: w430 -> [w431 w433]
      tunnel: [w431 w432] -> w428
      frame False {
      }
      frame True {
        n183 = call <vilib>:"Get File Extension.vi"("file"=w433) -> ("filename without extension"=w437:string, "lowercase file extension"=w434:string)  [unwired: 1 in, 8 out]
        n184 = Match Pattern(string=w437, regular expression="_") -> (before substring=w439:string, match substring=w438:string, after substring=w446:string)  [unwired: 2 out]
        n185 = Decimal String To Number(string=w446) -> (number=w444:i32)  [unwired: 3 out]
        n186 = Increment(x=w444) -> (x+1=w445:i32)
        n187 = Strip Path(path=w433) -> (stripped path=w442:path)  [unwired: 1 out]
        n188 = Path To String(path=w442) -> (string=w441:string)
        n189 = Number To Decimal String(number=w445) -> (decimal integer string=w436:string)  [unwired: 1 out]
        n190 = Concatenate Strings(w441, "\\" ("string"), w439, w438, w436, "." ("string"), w434) -> (w443:string)
        n191 = String To Path(string=w443) -> (path=w432:path)
      }
    }
    n192 = call <vilib>:"Check if File or Folder Exists.vi"("path"=w428) -> ("file or folder exists?"=w427:bool)  [unwired: 1 in, 9 out]
    n193 = Not(x=w427) -> (.not. x?=w426:bool)
  }
  n194 = call-poly <vilib>:"DAQmx Create Virtual Channel.vi"("physical channels"="AI Channels") -> ("task out"=w8:refnum<k21>)  [unwired: 8 in, 6 out]
  n195 = call-poly <vilib>:"DAQmx Timing.vi"("task/channels in"=w8, "sample mode"=w10, "samples per channel"="Buffer Size", "rate"="Sampling Rate") -> ("task out"=w6:refnum<k21>)  [unwired: 3 in, 8 out]
  n196 = call-poly <vilib>:"DAQmx Create Virtual Channel.vi"("lines"="Vid  Synch") -> ("task out"=w1:refnum<k21>)  [unwired: 6 in, 8 out]
  n197 = while {
    tunnel: w6 -> [w473]
    tunnel: w4 -> [w462]
    tunnel: w1 -> [w452]
    stop <- "stop" stop-if-true
    n198 = call-poly <vilib>:"DAQmx Read.vi"("task/channels in"=w473) -> ("data"=w472:waveform(dbl)[])  [unwired: 2 in, 12 out]
    n199 = call "Convert to Dynamic Data"("Array of Waveforms"=w472) -> ("Dynamic Data Type"=w461:dynamicdata)  [unwired: 3 out]
    n200 = Split Signals(w461) -> (w463:dynamicdata, w466:dynamicdata, w460:dynamicdata, w459:dynamicdata, →"EEG Chart":dynamicdata, w448:dynamicdata)  [unwired: 6 out]
    n201 = Merge Signals(w460, w459, w448) -> (→"Stimulation Chart":dynamicdata)
    n202 = Merge Signals(w463, w466) -> (→"DLM Chart":dynamicdata)
    n203 = case shown="True" "Show Triggered Response" {
      tunnel: w461 -> [_ w490]
      frame False {
      }
      frame True {
        n204 = call "Trigger and Gate"("Signals"=w490) -> ("Previous Signals"=w494:dynamicdata)  [unwired: 4 in, 6 out]
        n205 = Split Signals(w494) -> (w493:dynamicdata, w492:dynamicdata, w489:dynamicdata)  [unwired: 7 out]
        n206 = Merge Signals(w493, w492, w489) -> (→"Waveform Graph":dynamicdata)
      }
    }
    n207 = call <vilib>:"Boolean Crossing PtByPt.vi"("direction"=enum16{"either", "false-true", "true-false"}."true-false", "input"="Record") -> ("crossing"=w467:bool)  [unwired: 1 in]
    n208 = call "Write To Measurement File"("Signals"=w461, "Enable"="Record", "File Name"=w462) -> ("File Name Out"=w468:path, "Saving Data"=→"Recording":bool)  [unwired: 4 in, 11 out]
    "Trace File" <- w468
    n209 = call <vilib>:"Boolean Crossing PtByPt.vi"("initialize"=FALSE, "direction"=enum16{"either", "false-true", "true-false"}."false-true", "input"="Record") -> ("crossing"=w453:bool)
    n210 = And(x=w453, y="Vid Synch") -> (x .and. y?=w454:bool)
    n211 = case shown="True" w454 {
      tunnel: w452 -> [_ w478]
      frame False {
      }
      frame True {
        n212 = for {
          N: 5 -> [_]
          tunnel: w478 -> [w480]
          n213 = flat-sequence {
            tunnel: [w484] -> w481
            tunnel: w480 -> [w482]
            tunnel: w481 -> [w486]
            frame #0 {
              n214 = call-poly <vilib>:"DAQmx Write.vi"("task/channels in"=w482, "data"=TRUE) -> ("task out"=w484:refnum<k21>)  [unwired: 2 in, 11 out]
              n215 = Wait (ms)(milliseconds to wait=u32 100) -> ()  [unwired: 1 out]
            }
            frame #1 {
              n216 = call-poly <vilib>:"DAQmx Write.vi"("task/channels in"=w486, "data"=FALSE) -> ()  [unwired: 2 in, 12 out]
              n217 = Wait (ms)(milliseconds to wait=u32 100) -> ()  [unwired: 1 out]
            }
          }
        }
      }
    }
    n218 = case shown="False" "CoAx LED" {
      selector: "CoAx LED" -> [w474 w476]
      tunnel: w452 -> [w475 w477]
      frame False {
        n219 = call-poly <vilib>:"DAQmx Write.vi"("task/channels in"=w475, "data"=w474) -> ()  [unwired: 2 in, 12 out]
      }
      frame True {
        n220 = call-poly <vilib>:"DAQmx Write.vi"("task/channels in"=w477, "data"=w476) -> ()  [unwired: 2 in, 12 out]
      }
    }
    n221 = case shown="True" w467 {
      tunnel: w468 -> [_ w527]
      frame False {
      }
      frame True {
        n222 = local read "Puff Interval (s)"() -> (w495:dbl)
        n223 = local read "Sampling Rate"() -> (w504:dbl)
        n224 = local read "Train Duration (s)"() -> (w496:dbl)
        n225 = local read "Burst Dur (s)"() -> (w509:dbl)
        n226 = local read "Sound File"() -> (w500:path)
        n227 = local read "Burst Freq (Hz)"() -> (w513:dbl)
        n228 = local read "Test Dur (s)"() -> (w514:dbl)
        n229 = local read "Test Freq (Hz)"() -> (w515:dbl)
        n230 = Open/Create/Replace File(file path (use dialog)=w527, access (0:read/write)=enum16{"read/write", "read-only", "write-only"}."write-only") -> (refnum out=w521:refnum<file>)  [unwired: 1 in, 5 out]
        n231 = local read "Air Puff \nDuration (ms)"() -> (w497:u32)
        n232 = Get Date/Time In Seconds() -> (seconds since 1Jan1904=w517:timestamp)
        n233 = Format Date/Time String(time format string (%c)="%x", seconds (now)=w517) -> (date/time string=w511:string)  [unwired: 1 out]
        n234 = Format Date/Time String(time format string (%c)="%X", seconds (now)=w517) -> (date/time string=w510:string)  [unwired: 1 out]
        n235 = Path To String(path=w500) -> (string=w498:string)
        n236 = Set File Position(offset (in bytes) (0)=i64 0, refnum=w521, from (0:start)=enum16{"start", "end", "current"}."end") -> (refnum out=w522:refnum<file>)  [unwired: 1 in, 1 out]
        n237 = call "Build Text"("operator"="Operator", "date"=w511, "time"=w510, "genotype"="Genotype", "sex"="Sex", "age"="Age", "lineID"="Line ID", "pulse amplitude"="Pulse Amp. (V)", "test freq"=w515, "test duration"=w514, "burst freq"=w513, "burst duration"=w509, "sample rate"=w504, "Ch 1 name"="Ch 1. Name/Disc", "Ch 2 name"="Ch 2. Name/Disc", "Ch 3 name"="Ch 3. Name/Disc", "Mic FILENAME"=w498, "Air Puff Duration"=w497, "Air Puff Interval"=w495, "Air Train Duration"=w496, "Comments"="Comments") -> ("Result"=w520:string)  [unwired: 2 in, 4 out]
        n238 = Write to Text File(file (use dialog)=w522, text=w520) -> (refnum out=w526:refnum<file>)  [unwired: 1 in, 3 out]
        n239 = Close File(refnum=w526) -> ()  [unwired: 1 in, 2 out]
      }
    }
  }
  n240 = case shown="True" "Record Sound" {
    tunnel: w4 -> [_ w530]
    frame False {
    }
    frame True {
      w544 = T3 {"sample rate (S/s)"=22050.0, "number of channels"=2, "bits per sample"=16} ("Sound Format")
      w548 = T4 1 items=["Finite Samples", "Continuous Samples"] ("sample mode")
      # "4."
      # "2."
      # "1."
      n241 = Strip Path(path=w530) -> (stripped path=w537:path)  [unwired: 1 out]
      n242 = call <vilib>:"Get File Extension.vi"("file"=w530) -> ("filename without extension"=w534:string)  [unwired: 1 in, 9 out]
      n243 = Path To String(path=w537) -> (string=w536:string)
      n244 = Concatenate Strings(w536, "\\" ("string"), w534, "." ("string"), "wav" ("string")) -> (w531:string)
      n245 = String To Path(string=w531) -> (path=w529:path)
      "Sound File" <- w529
      n246 = call-poly <vilib>:"Sound File Open.vi"("sound format"=w544, "path"=w529) -> ("error out"=w546:errorcluster, "sound file refnum"=w542:T5)  [unwired: 1 in, 7 out]
      n247 = call <vilib>:"Sound Input Configure.vi"("number of samples/ch"=10000 ("Number of Samples/ch"), "sample mode"=w548, "error in (no error)"=w546, "sound format"=w544, "device ID"="Mic Ch") -> ("error out"=w538:errorcluster, "task ID"=w543:T6)  [unwired: 1 in, 4 out]
      n248 = while {
        shift-right: [w560] -> w539
        shift-left: w543 -> [w561]
        shift-right: [w559] -> w541
        shift-left: w542 -> [w558]
        shift-right: [w557] -> w540
        shift-left: w538 -> [w556]
        stop <- w554 stop-if-true
        # "3."
        n249 = call-poly <vilib>:"Sound Input Read.vi"("error in (no error)"=w556, "task ID"=w561) -> ("error out"=w562:errorcluster, "data"=w552:waveform(dbl)[], "task ID out"=w560:T6)  [unwired: 2 in, 5 out]
        n250 = local read "Record"() -> (w555:bool)
        n251 = local read "stop"() -> (w554:bool)
        n252 = case shown="True" w555 {
          tunnel: w562 -> [w563 w569]
          tunnel: w552 -> [_ w568]
          tunnel: [w564 w567] -> w559
          tunnel: w558 -> [w564 w566]
          tunnel: [w563 w565] -> w557
          frame False {
          }
          frame True {
            n253 = call-poly <vilib>:"Sound File Write.vi"("error in (no error)"=w569, "data"=w568, "sound file refnum"=w566) -> ("error out"=w565:errorcluster, "sound file refnum out"=w567:T5)  [unwired: 7 out]
          }
        }
        n254 = call-poly <vilib>:"FFT Power Spectral Density.vi"("averaging parameters"=T2 {"averaging mode"=enum."RMS averaging", "weighting mode"=enum."Exponential", "number of averages"=10}, "dB On (F)"=FALSE, "time signals"=w552) -> ("power spectral densities"=→"Microphone Periodogram":cluster{"f0":dbl, "df":dbl, "magnitude":dbl[]}[])  [unwired: 3 in, 5 out]
      }
      n255 = call <vilib>:"Sound Input Clear.vi"("error in (no error)"=w540, "task ID"=w539) -> ("error out"=w547:errorcluster)  [unwired: 9 out]
      n256 = call <vilib>:"Sound File Close.vi"("error in (no error)"=w547, "sound file refnum"=w541) -> ("error out"=w545:errorcluster)  [unwired: 9 out]
      n257 = call <vilib>:"Simple Error Handler.vi"("error in (no error)"=w545) -> ()  [unwired: 1 in, 8 out]
    }
  }
